vi "measure_j-v_keithley-2400.vi"(0 "User Name":string, 1 "Cell details cluster":T2={"Cell Position"=16, "Cell Label"="", "Pixel to measure"=0, "Area (cm^2)"=0.126, "Variable"="", "Variable value"="", "Scan settings in queue"=0, "Light or dark"="", "Measurement type"=""} {"Pixel to measure" items=["All", "1", "2", "3", "4", "5", "6", "7", "8"]}, 3 "Date array":string[](array[string]), 5 "Experiment Title":string, 12 "Scan settings":T1={"J-V scan"=TRUE, "Start voltage (V)"=0.0, "End voltage (V)"=0.0, "Step voltage (V)"=1.4, "Scan both directions"=TRUE, "Inverted device structure"=FALSE, "Measurement delay (ms)"=10.0, "Measurement speed"=0, "Scan rate (V/s)"=0.0, "Stabilisation time (s)"=0.0, "Stabilisation mode"=0, "Stabilisation value (V or A) "=1.0, "Illumination"=0, "Stabilisation in the dark?"=FALSE, "Repeat light scans"=FALSE, "No. of repeat scans"=0.0, "Only repeat for best pixel"=1, "J-t scan"=FALSE, "J-t best pixel only"=7, "J-t start voltage (V)"=0.0, "J-t end voltage (V)"=1.4, "J-t step voltage (V)"=0.01, "Step time (s)"=0.7, "J-t scan both directions"=TRUE, "J-t inverted device structure"=FALSE, "J-t settling delay (s)"=0.0, "J-t measurement speed"=0, "J-t illumination"=2, "Max. power stabilisation"=FALSE, "Max power best pixel only"=1, "Max. power point tracker"=FALSE, "Vmp from J-V scan"=FALSE, "Max P stab. Specific voltage"=FALSE, "Vmp (V)"=1.0, "Stabilisation time step (s)"=1.0, "Total stabilisation time (s)"=100.0} {"J-t settling delay (s)" min=10.0; "J-t illumination" items=["Light only", "Dark only", "Light then dark", "Dark then light"]; "Measurement speed" items=["Fast", "Normal", "High accuracy"]; "Illumination" items=["Light only", "Dark only", "Light then dark", "Dark then light"]; "Only repeat for best pixel" items=["only for best pixel", "for best 2 pixels", "for best 3 pixels", "for best 4 pixels", "for best 5 pixels", "for best 6 pixels", "for best 7 pixels", "for all pixels"]; "No. of repeat scans" min=1.0 step=1.0; "Max power best pixel only" items=["only the best pixel", "the best 2 pixels", "the best 3 pixels", "the best 4 pixels", "the best 5 pixels", "the best 6 pixels", "the best 7 pixels", "all pixels"]; "J-t best pixel only" items=["only the best pixel", "the best 2 pixels", "the best 3 pixels", "the best 4 pixels", "the best 5 pixels", "the best 6 pixels", "the best 7 pixels", "all pixels"]; "J-t measurement speed" items=["Fast", "Normal", "High Accuracy"]; "Stabilisation mode" items=["V", "I"]; "Measurement delay (ms)" min=10.0}, 13 "VISA resource name":refnum<visa-resource-name>="GPIB1::24::INSTR", 14 "Skip pixel?":bool) -> (4 "JV Curve":cluster{"Y":dbl[], "Y":dbl[]}[](graph), 6 "File path for master log":path, 15 "Log Table":string[][](table))   [LabVIEW 2016]
uses:
  TypeDefs/scan_settings.ctl
  <instrlib>/Keithley 24XX/Public/Data/Read (Single Point).vi
  <instrlib>/Keithley 24XX/Keithley 24XX.lvlib
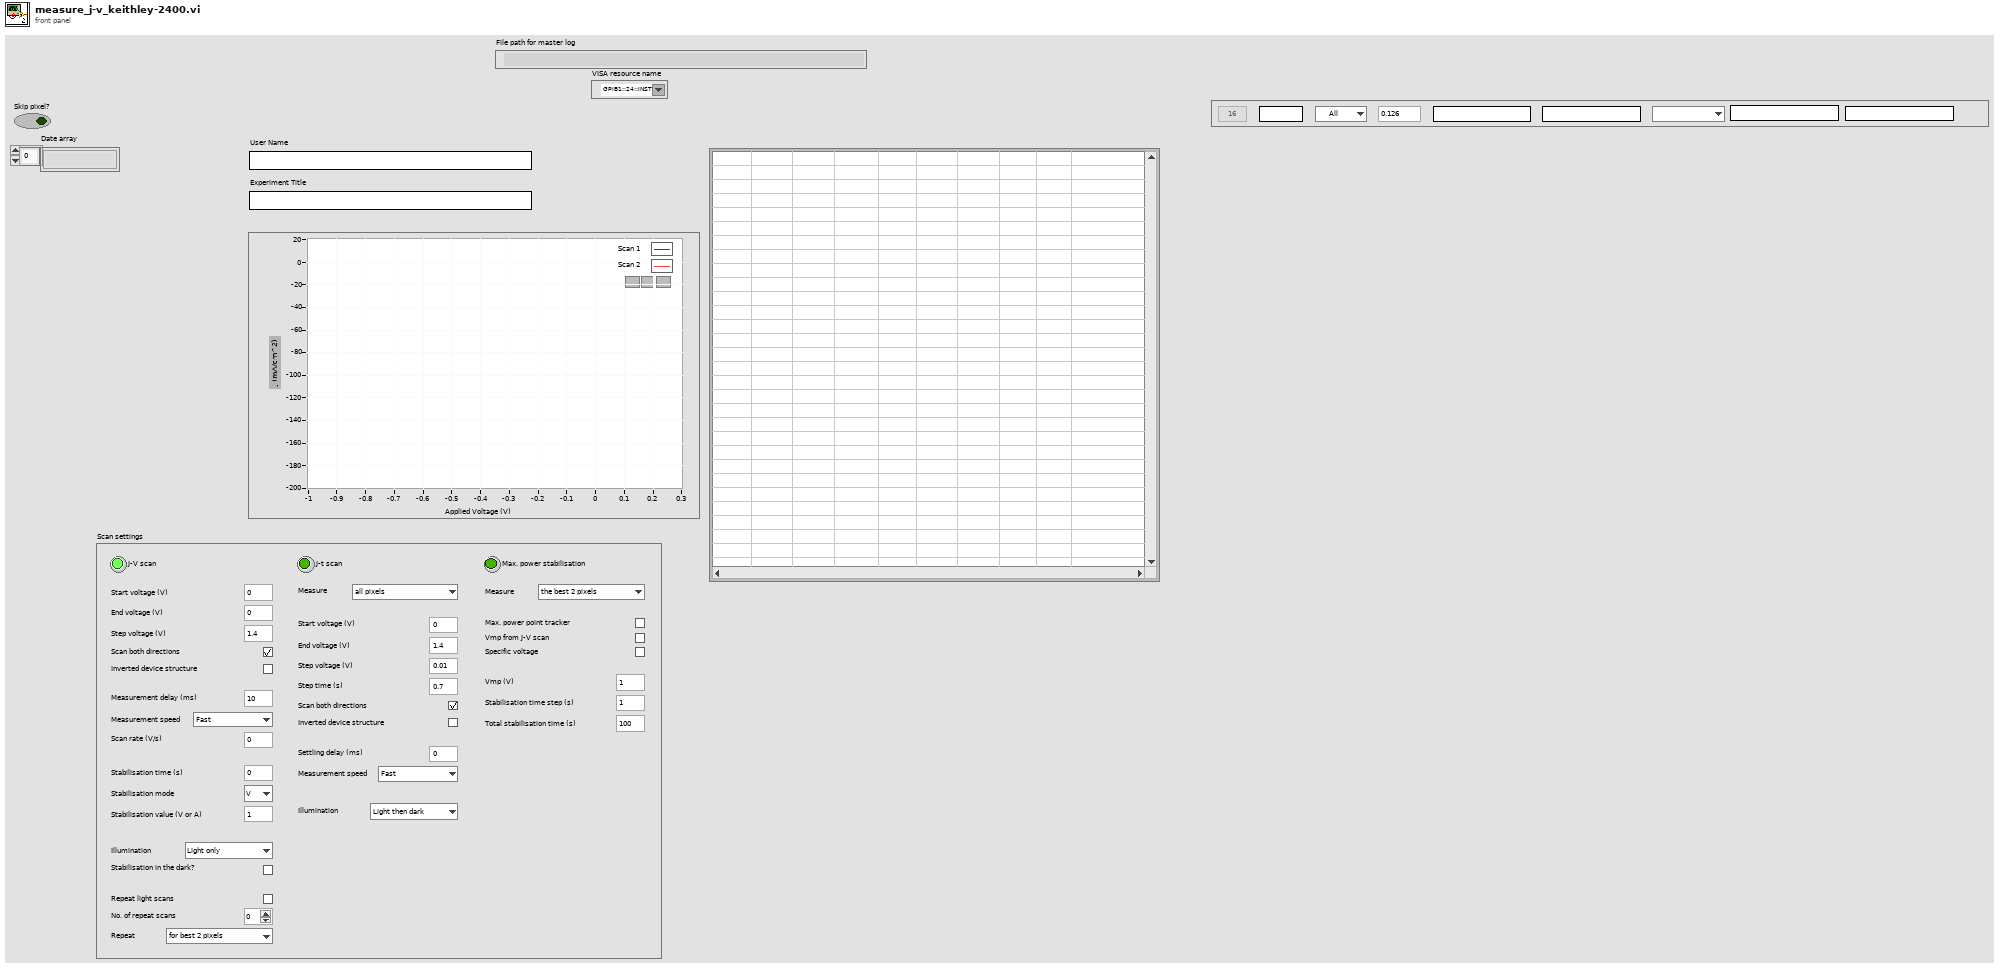
[diagram p1: front panel]
types:
  T1 = typedef "scan_settings.ctl" = cluster{"J-V scan":bool, "Start voltage (V)":dbl, "End voltage (V)":dbl, "Step voltage (V)":dbl, "Scan both directions":bool, "Inverted device structure":bool, "Measurement delay (ms)":dbl, "Measurement speed":u8, "Scan rate (V/s)":dbl, "Stabilisation time (s)":dbl, "Stabilisation mode":u16, "Stabilisation value (V or A) ":dbl, "Illumination":u16, "Stabilisation in the dark?":bool, "Repeat light scans":bool, "No. of repeat scans":dbl, "Only repeat for best pixel":u16, "J-t scan":bool, "J-t best pixel only":u16, "J-t start voltage (V)":dbl, "J-t end voltage (V)":dbl, "J-t step voltage (V)":dbl, "Step time (s)":dbl, "J-t scan both directions":bool, "J-t inverted device structure":bool, "J-t settling delay (s)":dbl, "J-t measurement speed":u16, "J-t illumination":u16, "Max. power stabilisation":bool, "Max power best pixel only":u16, "Max. power point tracker":bool, "Vmp from J-V scan":bool, "Max P stab. Specific voltage":bool, "Vmp (V)":dbl, "Stabilisation time step (s)":dbl, "Total stabilisation time (s)":dbl}
  T2 = cluster{"Cell Position":i32, "Cell Label":string, "Pixel to measure":u16, "Area (cm^2)":dbl, "Variable":string, "Variable value":string, "Scan settings in queue":u16, "Light or dark":string, "Measurement type":string}
  T3 = typedef "imagedata.ctl" = cluster{"image type":i32, "image depth":i32, "image":u8[], "mask":u8[], "colors":u32[], "Rectangle":cluster{"left":i16, "top":i16, "right":i16, "bottom":i16}}
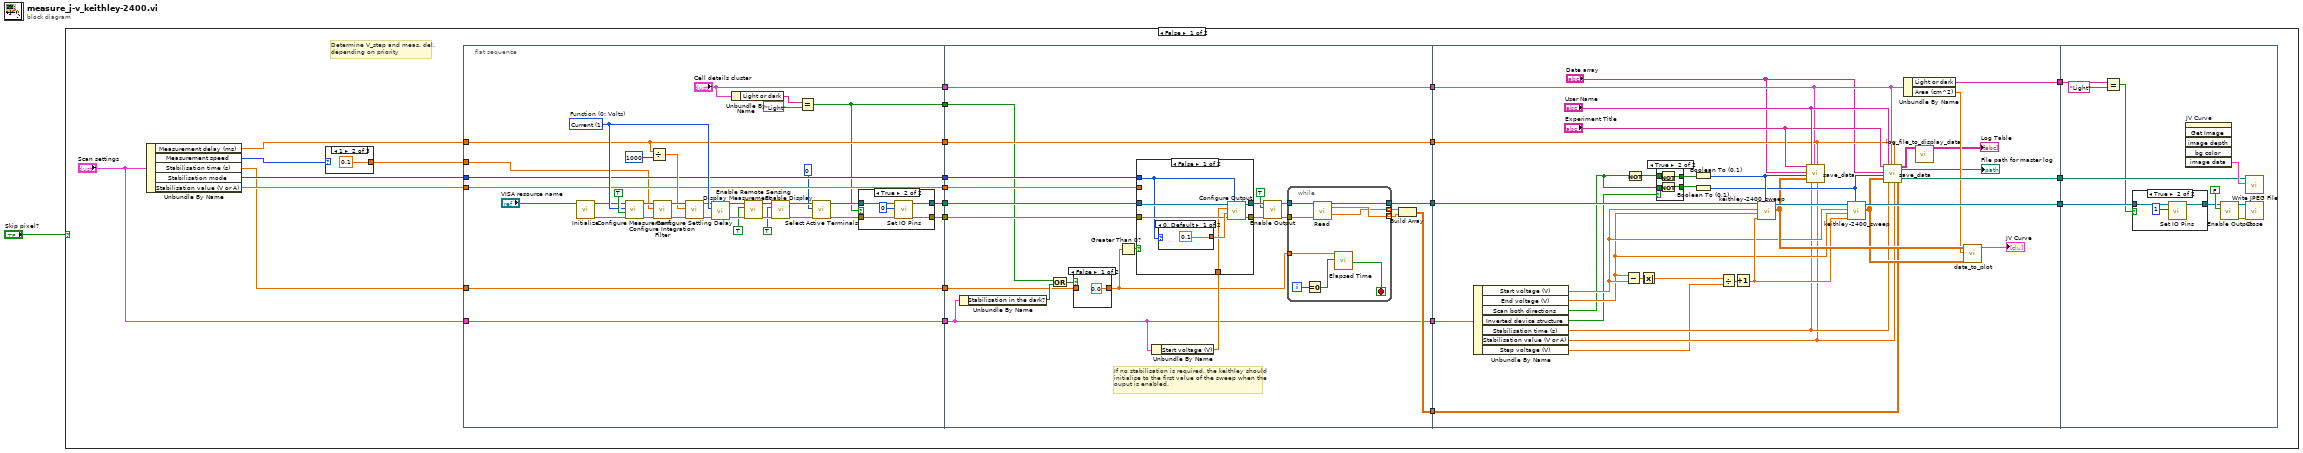
[diagram p0: block diagram]
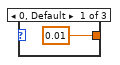
[diagram p2: hidden frame]
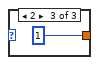
[diagram p3: hidden frame]
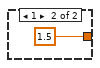
[diagram p6: hidden frame]
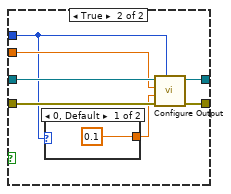
[diagram p7: hidden frame]
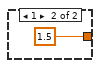
[diagram p8: hidden frame]
diagram:
  n1 = case shown="False" "Skip pixel?" {
    frame False {
      # "Determine V_step and meas. del.\ndepending on priority"
      n2 = Unbundle By Name("Scan settings") -> ("Measurement delay (ms)"=w2:dbl, "Measurement speed"=w3:u8, "Stabilisation time (s)"=w5:dbl, "Stabilisation mode"=w7:u16, "Stabilisation value (V or A)"=w8:dbl)
      n3 = case shown="1" w3 {
        tunnel: [0.01 0.1 1] -> w4
        frame 0, Default {
        }
        frame 1 {
        }
        frame 2 {
        }
      }
      n4 = flat-sequence {
        tunnel: [w46] -> w25
        tunnel: [w39] -> w24
        tunnel: [w40] -> w23
        tunnel: w8 -> [w46]
        tunnel: [w45] -> w22
        tunnel: w7 -> [w45]
        tunnel: [w44] -> w21
        tunnel: w5 -> [w44]
        tunnel: w2 -> [w43]
        tunnel: [w43] -> w20
        tunnel: [w42] -> w19
        tunnel: "Scan settings" -> [w42]
        tunnel: ["Cell details cluster"] -> w18
        tunnel: [w31] -> w17
        tunnel: w4 -> [w29]
        tunnel: w25 -> [w83]
        tunnel: w24 -> [w91]
        tunnel: w23 -> [w92]
        tunnel: [w87] -> w16
        tunnel: [w84] -> w15
        tunnel: w22 -> [w80]
        tunnel: w21 -> [w72]
        tunnel: [w82] -> w14
        tunnel: w20 -> [w82]
        tunnel: [w77] -> w13
        tunnel: w19 -> [w77]
        tunnel: [w81] -> w12
        tunnel: w18 -> [w81]
        tunnel: w17 -> [w75]
        tunnel: [w151] -> w11
        tunnel: [w144] -> w10
        tunnel: w16 -> [w158]
        tunnel: w15 -> [w143]
        tunnel: w14 -> [w140]
        tunnel: w13 -> [w139]
        tunnel: w12 -> [w133]
        tunnel: [w132] -> w9
        tunnel: w11 -> [w169]
        tunnel: w10 -> [w170]
        tunnel: w9 -> [w165]
        frame #0 {
          w60 = u16 1 items=["Volts", "Current", "Resistance"]  # Function (0: Volts)
          n5 = call <instrlib>:"Initialize.vi"("VISA resource name"="VISA resource name") -> ("error out"=w50:errorcluster, "VISA resource name out"=w51:refnum<visa-resource-name>)  [unwired: 4 in, 5 out]
          n6 = call <instrlib>:"Configure Measurement.vi"("error in (no error)"=w50, "Enable Auto Range (T:Enable)"=TRUE, "Function (0: Volts)"=w60, "VISA resource name"=w51) -> ("error out"=w53:errorcluster, "VISA resource name out"=w52:refnum<visa-resource-name>)  [unwired: 6 in]
          n7 = Divide(x=w43, y=1000) -> (x/y=w59:dbl)
          n8 = call <instrlib>:"Configure Integration Filter.vi"("error in (no error)"=w53, "Measurement Speed (1 PLC)"=w29, "VISA resource name"=w52) -> ("error out"=w62:errorcluster, "VISA resource name out"=w61:refnum<visa-resource-name>)  [unwired: 7 in]
          n9 = call <instrlib>:"Configure Settling Delay.vi"("error in (no error)"=w62, "Manual Settling Delay (0 sec)"=w59, "VISA resource name"=w61) -> ("error out"=w57:errorcluster, "VISA resource name out"=w56:refnum<visa-resource-name>)  [unwired: 7 in]
          n10 = call <instrlib>:"Display Measurement.vi"("error in (no error)"=w57, "Displayed Measurement (0: Voltage)"=w60, "VISA resource name"=w56) -> ("error out"=w55:errorcluster, "VISA resource name out"=w54:refnum<visa-resource-name>)  [unwired: 7 in]
          n11 = Unbundle By Name("Cell details cluster") -> ("Light or dark"=w38:string)
          n12 = call <instrlib>:"Enable Remote Sensing.vi"("error in (no error)"=w55, "Enable Remote Sensing (T: Enable)"=TRUE ("Enable Output (T: Enable)"), "VISA resource name"=w54) -> ("error out"=w48:errorcluster, "VISA resource name out"=w49:refnum<visa-resource-name>)  [unwired: 7 in]
          n13 = call <instrlib>:"Enable Display.vi"("error in (no error)"=w48, "Enable Display (T: Enable)"=TRUE, "VISA resource name"=w49) -> ("error out"=w35:errorcluster, "VISA resource name out"=w36:refnum<visa-resource-name>)  [unwired: 7 in]
          n14 = Equal?(x=w38, y="Light") -> (x = y?=w31:bool)
          n15 = call <instrlib>:"Select Active Terminals.vi"("error in (no error)"=w35, "Active Terminals (0: Front)"=0, "VISA resource name"=w36) -> ("error out"=w33:errorcluster, "VISA resource name out"=w34:refnum<visa-resource-name>)  [unwired: 7 in]
          n16 = case shown="True" w31 {
            tunnel: w34 -> [w66 w70]
            tunnel: w33 -> [w65 w69]
            tunnel: [w66 w68] -> w40
            tunnel: [w65 w67] -> w39
            frame False {
            }
            frame True {
              n17 = call <instrlib>:"Set IO Pins.vi"("error in (no error)"=w69, "Output Pattern (0)"=0, "VISA resource name"=w70) -> ("error out"=w67:errorcluster, "VISA resource name out"=w68:refnum<visa-resource-name>)  [unwired: 7 in]
            }
          }
        }
        frame #1 {
          # "If no stabilisation is required, the keithley should\ninitialise to the first value of the sweep when the\nouput is enabled."
          n18 = Unbundle By Name(w77) -> ("Stabilisation in the dark?"=w76:bool)
          n19 = Or(x=w75, y=w76) -> (x .or. y?=w74:bool)
          n20 = case shown="False" w74 {
            tunnel: [0.0 ("Stabilisation time (s)") w96] -> w73
            tunnel: w72 -> [_ w96]
            frame False {
            }
            frame True {
            }
          }
          n21 = Greater Than 0?(x=w73) -> (x > 0?=w79:bool)
          n22 = Unbundle By Name(w77) -> ("Start voltage (V)"=w78:dbl)
          n23 = case shown="False" w79 {
            tunnel: [w101 w112] -> w94
            tunnel: [w102 w111] -> w93
            tunnel: w92 -> [w99 w110]
            tunnel: w91 -> [w100 w109]
            tunnel: w83 -> [_ w108]
            tunnel: w80 -> [w98 w107]
            tunnel: w78 -> [w97 _]
            frame False {
              n24 = case shown="0, Default" w98 {
                tunnel: [0.1 1.5] -> w103
                frame 0, Default {
                }
                frame 1 {
                }
              }
              n25 = call <instrlib>:"Configure Output.vi"("Source Mode  (0: Voltage)"=w98, "error in (no error)"=w100, "Compliance  Level (0.1)"=w103, "Output Level (0)"=w97, "VISA resource name"=w99) -> ("error out"=w101:errorcluster, "VISA resource name out"=w102:refnum<visa-resource-name>)  [unwired: 5 in]
            }
            frame True {
              n26 = case shown="0, Default" w107 {
                tunnel: [0.1 1.5] -> w106
                frame 0, Default {
                }
                frame 1 {
                }
              }
              n27 = call <instrlib>:"Configure Output.vi"("Source Mode  (0: Voltage)"=w107, "error in (no error)"=w109, "Compliance  Level (0.1)"=w106, "Output Level (0)"=w108, "VISA resource name"=w110) -> ("error out"=w112:errorcluster, "VISA resource name out"=w111:refnum<visa-resource-name>)  [unwired: 5 in]
            }
          }
          n28 = call <instrlib>:"Enable Output.vi"("error in (no error)"=w94, "Enable Output (T: Enable)"=TRUE ("Output (Off)"), "VISA resource name"=w93) -> ("error out"=w88:errorcluster, "VISA resource name out"=w89:refnum<visa-resource-name>)  [unwired: 7 in]
          n29 = while {
            tunnel: w89 -> [w123]
            tunnel: w88 -> [w122]
            tunnel: [w121] -> w87
            tunnel: [w115] -> w86 mode=indexing
            tunnel: [w119] -> w85 mode=indexing
            tunnel: w73 -> [w116]
            i -> [w118]
            stop <- w120 stop-if-true
            n30 = Equal To 0?(x=w118) -> (x = 0?=w117:bool)
            n31 = call-poly <instrlib>:"Read.vi"("VISA resource name"=w123, "error in (no error)"=w122) -> ("VISA resource name out"=w121:refnum<visa-resource-name>, "Current"=w119:sgl, "Timestamp"=w115:sgl)  [unwired: 7 in, 4 out]
            n32 = call "Elapsed Time"("Time Target (s)"=w116, "Reset"=w117) -> ("Time has Elapsed"=w120:bool)  [unwired: 10 in, 7 out]
          }
          n33 = Build Array(w86, w85) -> (w84:sgl[][])
        }
        frame #2 {
          n34 = Unbundle By Name(w139) -> ("Start voltage (V)"=w138:dbl, "End voltage (V)"=w137:dbl, "Scan both directions"=w127:bool, "Inverted device structure"=w136:bool, "Stabilisation time (s)"=w135:dbl, "Stabilisation value (V or A)"=w134:dbl, "Step voltage (V)"=w124:dbl)
          n35 = Subtract(x=w137, y=w138) -> (x-y=w156:dbl)
          n36 = Not(x=w127) -> (.not. x?=w128:bool)
          n37 = Absolute Value(x=w156) -> (abs(x)=w157:dbl)
          n38 = case shown="True" w136 {
            tunnel: [w160 w164] -> w146
            tunnel: [w159 w163] -> w145
            tunnel: w127 -> [w159 w162]
            tunnel: w128 -> [w160 w161]
            frame False {
            }
            frame True {
              n39 = Not(x=w161) -> (.not. x?=w164:bool)
              n40 = Not(x=w162) -> (.not. x?=w163:bool)
            }
          }
          n41 = Boolean To (0,1)(Boolean=w146) -> (0, 1=w154:i16)
          n42 = Boolean To (0,1)(Boolean=w145) -> (0, 1=w152:i16)
          n43 = Divide(x=w157, y=w124) -> (x/y=w148:dbl)
          n44 = Increment(x=w148) -> (x+1=w147:dbl)
          n45 = call "keithley-2400_sweep.vi"("Sweep Direction"=w154, "Number of Points"=w147, "Maximum Amplitude"=w137, "Minimum Amplitude"=w138, "VISA resource name out 2"=w158) -> ("Data Array"=w150:dbl[][], "VISA resource name out"=w153:refnum<visa-resource-name>)  [unwired: 2 in, 1 out]
          n46 = call "save_data.vi"("Experiment Indicator"="Experiment Title", "Date array"="Date array", "Scan direction"=w154, "Data Array"=w150, "Username"="User Name", "Stabilisation time (ms)"=w135, "Cell details cluster"=w133, "Measurement Delay (ms)"=w140, "Stabilisation level \n(A or V depending on mode)"=w134) -> ()  [unwired: 7 in, 4 out]
          n47 = call "keithley-2400_sweep.vi"("Sweep Direction"=w152, "Number of Points"=w147, "Maximum Amplitude"=w137, "Minimum Amplitude"=w138, "VISA resource name out 2"=w153) -> ("Data Array"=w149:dbl[][], "VISA resource name out"=w151:refnum<visa-resource-name>)  [unwired: 2 in, 1 out]
          n48 = call "save_data.vi"("Experiment Indicator"="Experiment Title", "Date array"="Date array", "Scan direction"=w152, "Data Array"=w149, "Username"="User Name", "Stabilisation time (ms)"=w135, "Cell details cluster"=w133, "Measurement Delay (ms)"=w140, "Stabilisation level \n(A or V depending on mode)"=w134, "Stabilisation Data"=w143) -> ("Master Log"=w130:string[][], "File path for master log"=→"File path for master log":path, "File path for JV image"=w144:path)  [unwired: 6 in, 1 out]
          n49 = Unbundle By Name(w133) -> ("Light or dark"=w132:string, "Area (cm^2)"=w131:dbl)
          n50 = call "log_file_to_display_data.vi"("Master Log"=w130) -> ("Formatted table"=→"Log Table":string[][])  [unwired: 10 in]
          n51 = call "data_to_plot.vi"("Data Array 2"=w149, "Device Area (cm^2)"=w131, "Data Array"=w150) -> ("JV Curve"=→"JV Curve":cluster{"Y":dbl[], "Y":dbl[]}[])  [unwired: 8 in]
        }
        frame #3 {
          n52 = Equal?(x=w165, y="Light") -> (x = y?=w166:bool)
          n53 = case shown="True" w166 {
            tunnel: w169 -> [w175 w177]
            tunnel: [w175 w176] -> w168
            frame False {
            }
            frame True {
              n54 = call <instrlib>:"Set IO Pins.vi"("Output Pattern (0)"=1, "VISA resource name"=w177) -> ("VISA resource name out"=w176:refnum<visa-resource-name>)  [unwired: 8 in, 1 out]
            }
          }
          n55 = invoke on="JV Curve" class="XYGraph (strict)" method="Get Image"() -> ("image data"=w171:T3)  [unwired: 6 in, 5 out]
          n56 = call <instrlib>:"Enable Output.vi"("Enable Output (T: Enable)"=FALSE ("Output (Off)"), "VISA resource name"=w168) -> ("error out"=w173:errorcluster, "VISA resource name out"=w174:refnum<visa-resource-name>)  [unwired: 8 in]
          n57 = call <vilib>:"Write JPEG File.vi"("image data"=w171, "path to JPEG file"=w170) -> ()  [unwired: 8 in, 2 out]
          n58 = call <instrlib>:"Close.vi"("error in (no error)"=w173, "VISA resource name"=w174) -> ()  [unwired: 9 in, 1 out]
        }
      }
    }
    frame True {
    }
  }
